vi "Init.vi"(5 "Bus In":refnum<class "Bus.lvclass">, 7 "Scaling Cluster":T1, 8 "error in (no error)":errorcluster, 9 "Init or Array":bool, 10 "Array":dbl[](array[numeric]), 11 "All Channels in":refnum<class "All Channels Out.lvclass">) -> (0 "error out":errorcluster, 2 "Bus Out":refnum<class "Bus.lvclass">, 3 "All Channels out":refnum<class "All Channels Out.lvclass">)   [LabVIEW 2018, in "All Channels Out.lvclass"]
uses:
  All Channels Out.lvclass
  Scaling/Scaling.lvclass
  Bus/Bus.lvclass
  All Channels Out.lvclass/All Channels Out.ctl
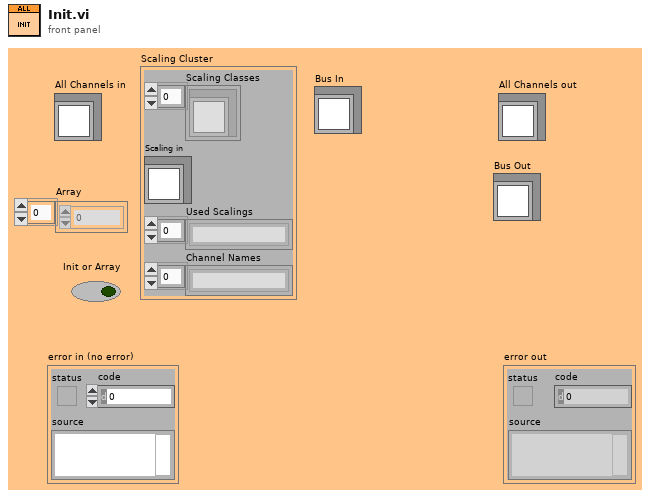
[diagram p1: front panel]
types:
  T1 = cluster{"Scaling Classes":refnum<class "Scaling.lvclass">[], "Scaling in":refnum<class "Scaling.lvclass">, "Used Scalings":string[], "Channel Names":string[]}
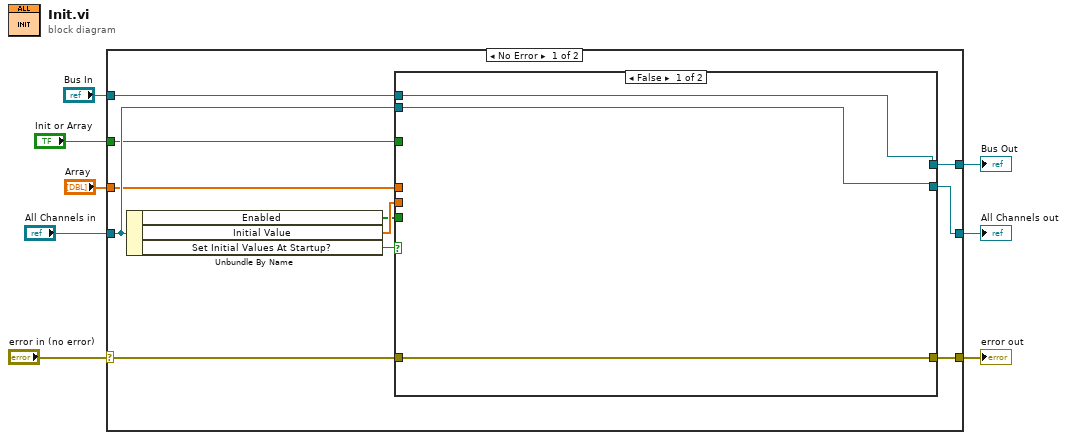
[diagram p0: block diagram]
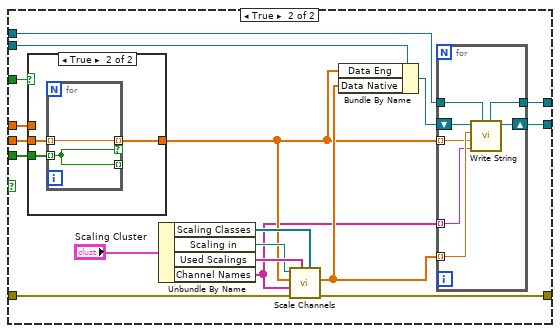
[diagram p2: hidden frame]
diagram:
  n1 = case shown="No Error" "error in (no error)" {
    selector: "error in (no error)" -> [w14 w59]
    tunnel: [w13 w59] -> w7
    tunnel: [w12 w60] -> w6
    tunnel: "All Channels in" -> [w19 w60]
    tunnel: "Init or Array" -> [w18 _]
    tunnel: "Array" -> [w16 _]
    tunnel: [w11 w58] -> w2
    tunnel: "Bus In" -> [w10 w58]
    frame No Error {
      n2 = Unbundle By Name(w19) -> ("Enabled"=w15:bool[], "Initial Value"=w17:dbl[], "Set Initial Values At Startup?"=w9:bool)
      n3 = case shown="False" w9 {
        tunnel: w19 -> [w21 w40]
        tunnel: w18 -> [_ w39]
        tunnel: w17 -> [_ w38]
        tunnel: w16 -> [_ w37]
        tunnel: w15 -> [_ w36]
        tunnel: w14 -> [w20 w31]
        tunnel: [w20 w30] -> w13
        tunnel: [w21 w29] -> w12
        tunnel: [w22 w24] -> w11
        tunnel: w10 -> [w22 w23]
        frame False {
        }
        frame True {
          n4 = case shown="True" w39 {
            tunnel: w38 -> [_ w54]
            tunnel: [w48 w53] -> w26
            tunnel: w37 -> [w49 _]
            tunnel: w36 -> [w50 w55]
            frame False {
              n5 = for {
                tunnel: [w51] -> w48 mode=indexing if=w52
                tunnel: w50 -> [w52] mode=indexing
                tunnel: [w52] -> _ mode=indexing
                tunnel: w49 -> [w51] mode=indexing
              }
            }
            frame True {
              n6 = for {
                tunnel: [w56] -> w53 mode=indexing if=w57
                tunnel: w55 -> [w57] mode=indexing
                tunnel: [w57] -> _ mode=indexing
                tunnel: w54 -> [w56] mode=indexing
              }
            }
          }
          n7 = Unbundle By Name("Scaling Cluster") -> ("Scaling Classes"=w33:refnum<class "Scaling.lvclass">[], "Scaling in"=w34:refnum<class "Scaling.lvclass">, "Used Scalings"=w35:string[], "Channel Names"=w25:string[])
          n8 = call "Scale Channels.vi"("Scaling Classes"=w33, "Used Scalings"=w35, "error in (no error)"=w31, "Channel Names"=w25, "Values In"=w26, "Scaling in"=w34) -> ("error out"=w30:errorcluster, "Values Out"=w27:dbl[])  [unwired: 3 in, 1 out]
          n9 = Bundle By Name(cluster=w40, "Data Eng"=w26, "Data Native"=w27) -> (w28:refnum<class "All Channels Out.lvclass">)
          n10 = for {
            tunnel: w27 -> [w45] mode=indexing
            tunnel: w26 -> [w44] mode=indexing
            shift-right: [w47] -> w29
            shift-left: w28 -> [w46]
            tunnel: w25 -> [w43] mode=indexing
            tunnel: [w42] -> w24
            tunnel: w23 -> [w41]
            n11 = call-dynamic "Write String.vi"("Bus In"=w41, "Channel Name"=w43, "Data Value Engineering"=w44, "Data Value Native"=w45, "All Channels in"=w46) -> ("All Channels out"=w47:refnum<class "All Channels Out.lvclass">, "Bus Out"=w42:refnum<class "Bus.lvclass">)  [unwired: 4 in, 1 out]
          }
        }
      }
    }
    frame Error {
    }
  }
  "error out" <- w7
  "All Channels out" <- w6
  "Bus Out" <- w2
